vi "TimeCalc.vi"(8 "Auto Common Settings":T1, 10 "Time Calc Cluster":T2) -> (3 "Time":dbl)   [LabVIEW 2017]
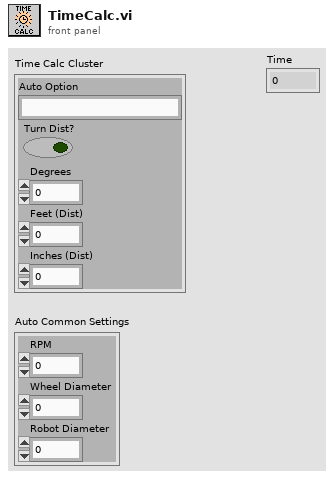
[diagram p1: front panel]
types:
  T1 = cluster{"RPM":dbl, "Wheel Diameter":dbl, "Robot Diameter":dbl}
  T2 = cluster{"Turn Dist?":bool, "Feet (Dist)":dbl, "Inches (Dist)":dbl, "Degrees":dbl, "Auto Option":string}
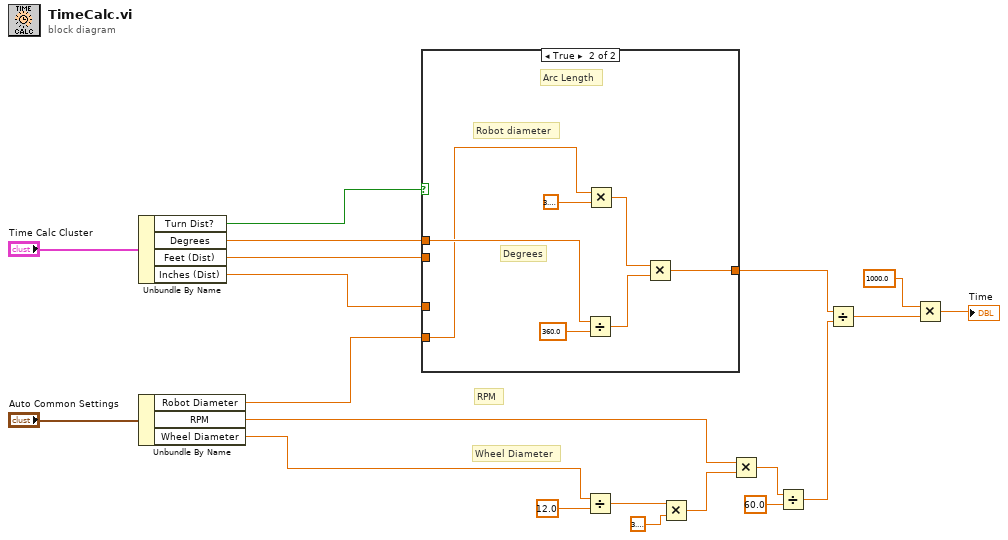
[diagram p0: block diagram]
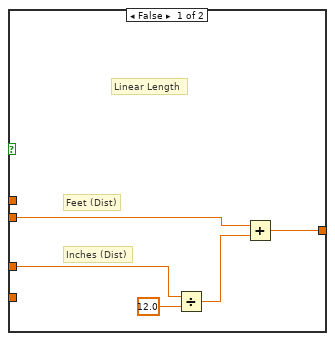
[diagram p2: hidden frame]
diagram:
  # "Wheel Diameter"
  # "RPM"
  n1 = Unbundle By Name("Time Calc Cluster") -> ("Turn Dist?"=w8:bool, "Degrees"=w7:dbl, "Feet (Dist)"=w6:dbl, "Inches (Dist)"=w5:dbl)
  n2 = Unbundle By Name("Auto Common Settings") -> ("Robot Diameter"=w1:dbl, "RPM"=w3:dbl, "Wheel Diameter"=w2:dbl)
  n3 = case shown="True" w8 {
    tunnel: [w23 w30] -> w13
    tunnel: w7 -> [_ w27]
    tunnel: w6 -> [w22 _]
    tunnel: w5 -> [w21 _]
    tunnel: w1 -> [_ w26]
    frame False {
      # "Inches (Dist)"
      # "Feet (Dist)"
      # "Linear Length"
      n4 = Divide(x=w21, y=12.0) -> (x/y=w24:dbl)
      n5 = Add(x=w22, y=w24) -> (x+y=w23:dbl)
    }
    frame True {
      # "Degrees"
      # "Robot diameter"
      # "Arc Length"
      n6 = Divide(x=w27, y=360.0) -> (x/y=w31:dbl)
      n7 = Multiply(x=w26, y=3.141592653589793) -> (x*y=w28:dbl)
      n8 = Multiply(x=w28, y=w31) -> (x*y=w30:dbl)
    }
  }
  n9 = Divide(x=w2, y=12.0) -> (x/y=w14:dbl)
  n10 = Multiply(x=w14, y=3.141592653589793) -> (x*y=w19:dbl)
  n11 = Multiply(x=w3, y=w19) -> (x*y=w18:dbl)
  n12 = Divide(x=w18, y=60.0) -> (x/y=w16:dbl)
  n13 = Divide(x=w13, y=w16) -> (x/y=w11:dbl)
  n14 = Multiply(x=1000.0, y=w11) -> (x*y=→"Time":dbl)
